vi "Resync_OpalRT_LC2.vi"() -> ()   [LabVIEW 2016]
uses:
  LabVIEW Data/MathScriptVIs/MCStatic_36913153632_439bfbade32b9795c282450b08103ccf.vi
  <instcachedir>/0/MCStatic_36913153632_439bfbade32b9795c282450b08103ccf_1263693CE67B40CA8D12AD81B2A866E4.lvgen/MCStatic_36913153632_439bfbade32b9795c282450b08103ccf_1263693CE67B40CA8D12AD81B2A866E4_003.vi
  <vilib>/imath/engines/lvmath2/RunTimeEngine/NodeEndStatement/NIMS_NodeEndStatement_Output.vi
  <instcachedir>/0/NIMS_NodeEndStatement_Output_53EC0D466D134D7ABD903AC30B43404B.lvgen/NIMS_NodeEndStatement_Output_53EC0D466D134D7ABD903AC30B43404B_001.vi
  <vilib>/imath/engines/lvmath2/RunTimeEngine/ErrorHandling/NIMS_Finalize Error.vi
  LCs_forRTDS/Dependencies/PIcontroller.m
panel:
  out "error out 2":errorcluster
  in  "i_an 2":dbl=0.09999999999999964
  in  "p_an 2":dbl=0.20000000000000018
  in  "i_in 2":dbl=4.1
  in  "p_in 2":dbl=3.0999999999999996
  in  "p_in":dbl=3.0999999999999996
  in  "i_in":dbl=4.1
  in  "p_an":dbl=0.20000000000000018
  in  "i_an":dbl=0.09999999999999964
  out "error out":errorcluster
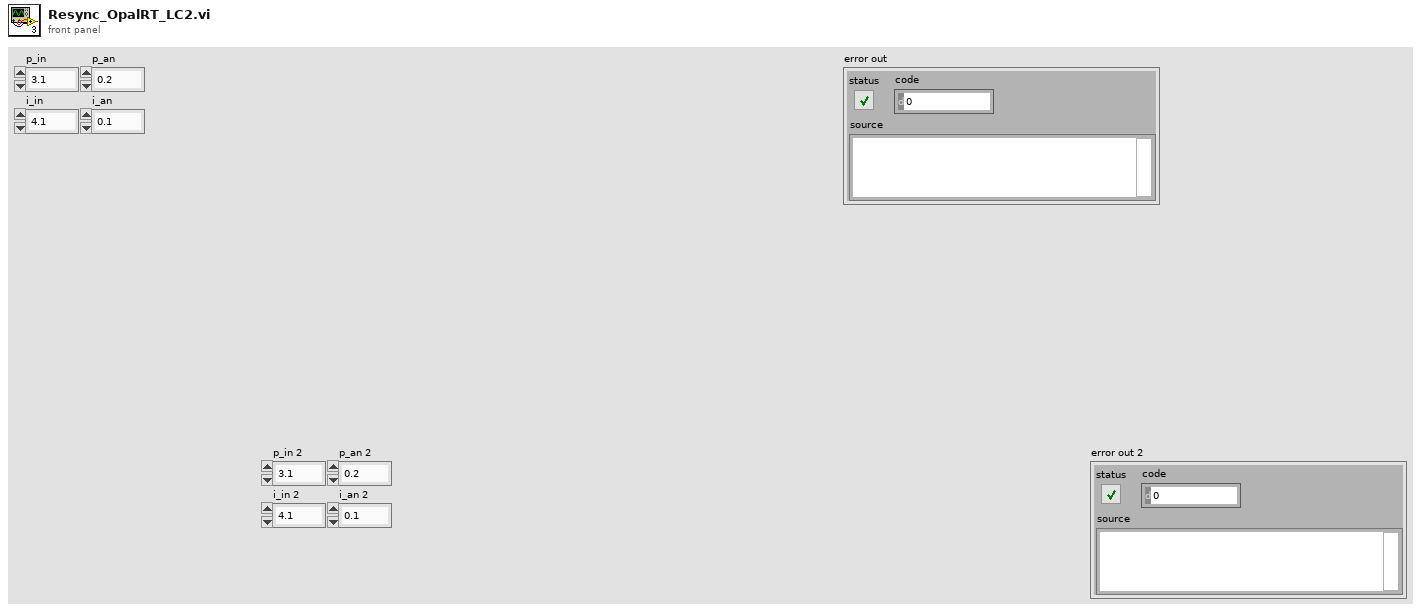
[diagram p1: front panel]
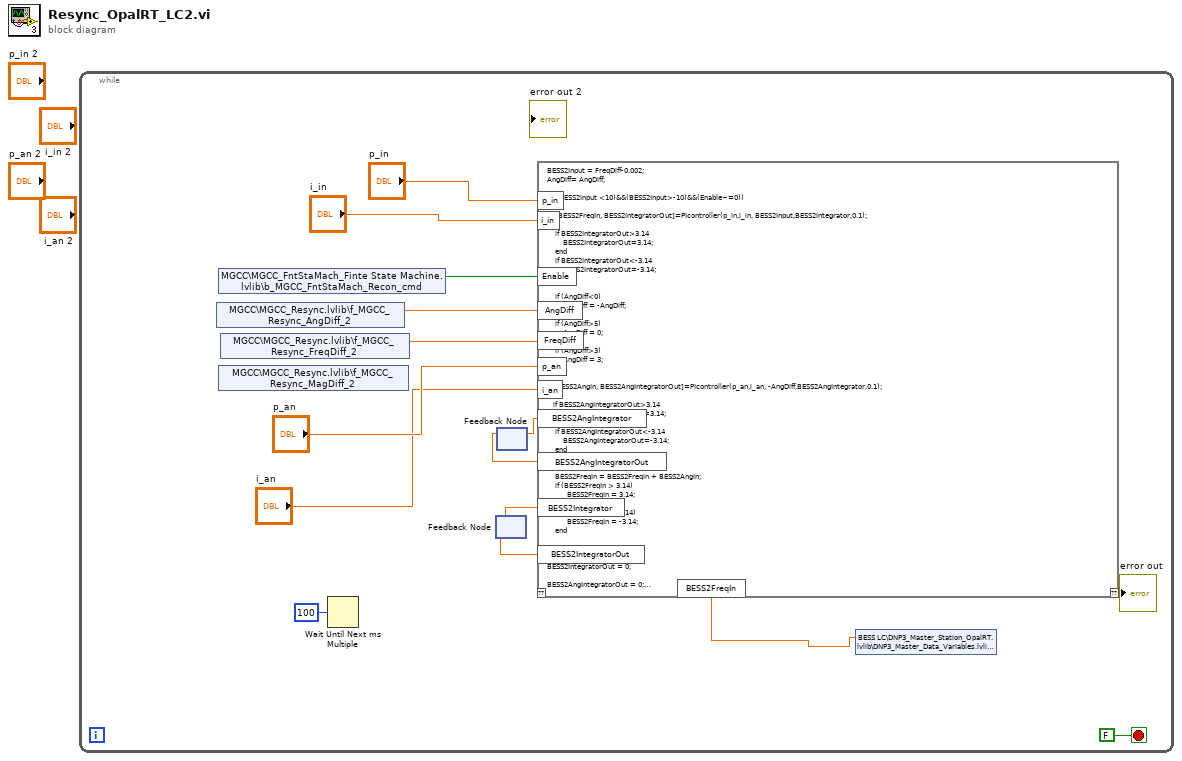
[diagram p0: block diagram]
diagram:
  n1 = while {
    stop <- FALSE stop-if-true
    n2 = shared-variable "MGCC\\MGCC_Resync.lvlib\\f_MGCC_Resync_AngDiff_2"() -> (w13:dbl)  [unwired: 1 in, 1 out]
    n3 = shared-variable "MGCC\\MGCC_FntStaMach_Finte State Machine.lvlib\\b_MGCC_FntStaMach_Recon_cmd"() -> (w9:bool)  [unwired: 1 in, 1 out]
    n4 = shared-variable "MGCC\\MGCC_Resync.lvlib\\f_MGCC_Resync_MagDiff_2"() -> ()  [unwired: 1 in, 2 out]
    n5 = shared-variable "MGCC\\MGCC_Resync.lvlib\\f_MGCC_Resync_FreqDiff_2"() -> (w12:dbl)  [unwired: 1 in, 1 out]
    n6 = Wait Until Next ms Multiple(millisecond multiple=u32 100) -> ()  [unwired: 1 out]
    n7 = feedback #1() -> (w15:dbl)  [unwired: 1 in]
    n8 = feedback #2() -> (w10:dbl)  [unwired: 1 in]
    n9 = mathscript code="BESS2Input = FreqDiff-0.002;\nAngDiff= AngDiff;\n\nif ((BESS2Input <10)&&(BESS2Input>-10)&&(Enable~=0))\n\n    [BESS2FreqIn, BESS2IntegratorOut]=PIcontroller(p_in,i_in, BESS2Input,BESS2Integrator,0.1);\n   \n    if BESS2IntegratorOut>3.14\n        BESS2IntegratorOut=3.14;\n    end\n    if BESS2IntegratorOut<-3.14\n        BESS2IntegratorOut=-3.14;\n    end\n\n    if (AngDiff<0)\n        AngDiff = -AngDiff;\n    end \n    if (AngDiff>5)\n        AngDiff = 0;\n    end \n    if (AngDiff>3)\n        AngDiff = 3;\n    end \n\n   [BESS2AngIn, BESS2AngIntegratorOut]=PIcontroller(p_an,i_an, -AngDiff,BESS2AngIntegrator,0.1);\n\n   if BESS2AngIntegratorOut>3.14\n        BESS2AngIntegratorOut=3.14;\n    end\n    if BESS2AngIntegratorOut<-3.14\n        BESS2AngIntegratorOut=-3.14;\n    end\n    \n\n    BESS2FreqIn = BESS2FreqIn + BESS2AngIn;\n    if (BESS2FreqIn > 3.14) \n          BESS2FreqIn = 3.14;\n    end\n    if (BESS2FreqIn < -3.14) \n          BESS2FreqIn = -3.14;\n    end\n\nelse\nBESS2FreqIn = 0;\nBESS2IntegratorOut = 0;\n\nBESS2AngIntegratorOut = 0;\nend"("AngDiff"=w13, "BESS2Integrator"=w15, "FreqDiff"=w12, "BESS2AngIntegrator"=w10, "Enable"=w9, "p_in"="p_in", "i_in"="i_in", "p_an"="p_an", "i_an"="i_an") -> ("??"=→"error out":errorcluster, "BESS2IntegratorOut"=w14:dbl, "BESS2FreqIn"=w6:dbl, "BESS2AngIntegratorOut"=w11:dbl)  [unwired: 1 in]
    n10 = feedback-in #1(w14) -> ()
    n11 = feedback-in #2(w11) -> ()
    n12 = shared-variable "BESS LC\\DNP3_Master_Station_OpalRT.lvlib\\DNP3_Master_Data_Variables.lvlib\\MS_Analog_Control.lvlib\\BESS2-FREQ-CMD"(w6) -> ()  [unwired: 1 in, 1 out]
  }
